vi "Initialize camera.vi"() -> (2 "CUDA device ID":i32, 3 "IMAQdx Session Out":T1, 4 "TrueFrame out":i32, 6 "IMAQ camera":bool, 8 "Image reference out":T2, 10 "SLM enabled":bool=TRUE, 11 "Camera enabled":bool=TRUE, 12 "Vision error out":errorcluster, 13 "LUT path out":path, 14 "IMAQ Session Out":refnum<k11>, 15 "Camera error":errorcluster)   [LabVIEW 2009]
uses:
  <vilib>/vision/Image Controls.llb/IMAQ Image.ctl
  <vilib>/userDefined/High Color/IMAQdx.ctl
  <vilib>/vision/driver/NI_Vision_Acquisition_Software.lvlib
panel:
  in  "CUDA device ID":i32
  in  "LUT file (full path)":path
  in  "TrueFrame":i32=6
  in  "Select camera type":u16(ring)=2 items=["IMAQ (Camera Link)", "IMAQdx (firewire)", "No camera"]
  in  "SLM enabled":bool
  in  "Start":bool
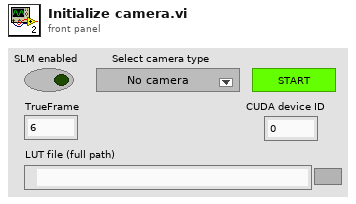
[diagram p1: front panel]
types:
  T1 = typedef "IMAQdx.ctl" = refnum<k21>
  T2 = typedef "IMAQ Image.ctl" = refnum<image>
  T3 = typedef "Image Type" = u32
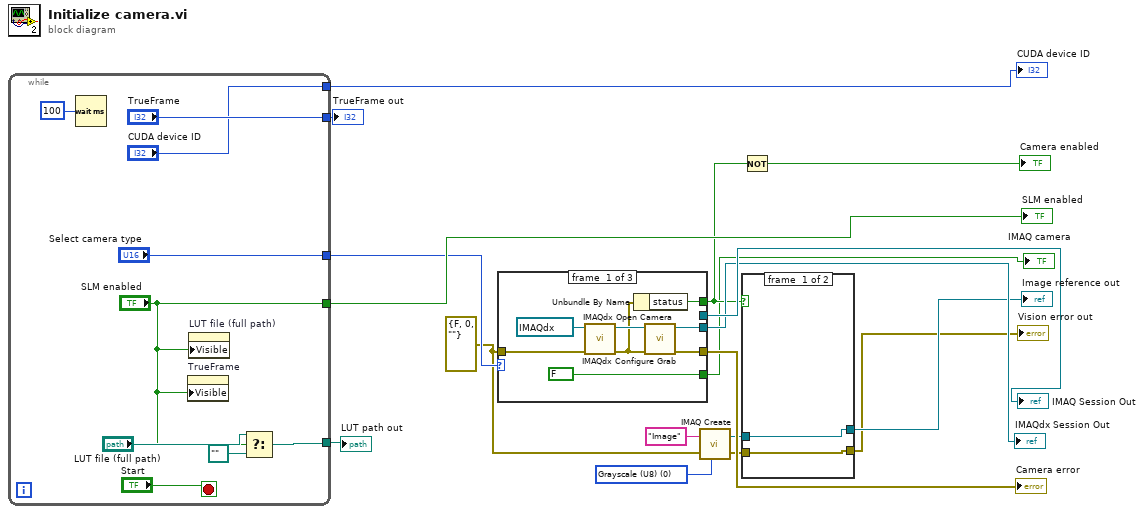
[diagram p0: block diagram]
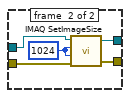
[diagram p2: hidden frame]
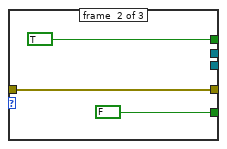
[diagram p3: hidden frame]
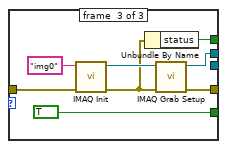
[diagram p4: hidden frame]
diagram:
  w8 = T3 0 items=["Grayscale (U8)", "Grayscale (I16)", "Grayscale (SGL)", "Complex (CSG)", "RGB (U32)", "HSL (U32)", "RGB (U64)", "Grayscale (U16)"] ("Image Type")
  w7 = errorcluster {"status"=FALSE, "code"=0, "source"=""} ("Camera error")
  n1 = while {
    tunnel: ["SLM enabled"] -> w16
    tunnel: ["Select camera type"] -> w12
    tunnel: ["TrueFrame"] -> w3
    tunnel: [w22] -> w2
    tunnel: ["CUDA device ID"] -> w1
    stop <- "Start" stop-if-true
    n2 = Wait (ms)(milliseconds to wait=u32 100) -> ()  [unwired: 1 out]
    n3 = property on="TrueFrame" class="DigNum (strict)"("Visible"="SLM enabled") -> ()  [unwired: 2 in, 2 out]
    n4 = property on="LUT file (full path)" class="Path"("Visible"="SLM enabled") -> ()  [unwired: 2 in, 2 out]
    n5 = Select(t="LUT file (full path)", s="SLM enabled", f=path "") -> (s? t:f=w22:path)
  }
  "SLM enabled" <- w16
  "TrueFrame out" <- w3
  "LUT path out" <- w2
  "CUDA device ID" <- w1
  n6 = case shown="2, Default" w12 {
    tunnel: [_ _ w44] -> w18
    tunnel: w7 -> [w35 w38 w43]
    tunnel: [w33 _ _] -> w17
    tunnel: [w30 TRUE ("status") w41] -> w11
    tunnel: [w29 w38 w40] -> w13
    tunnel: [FALSE ("IMAQ camera") FALSE ("IMAQ camera") TRUE ("IMAQ camera")] -> w10
    frame #0 {
      n7 = call <vilib>:"IMAQdx Open Camera.vi"("error in"=w35, "Session In"=T1 "cam0") -> ("error out"=w31:errorcluster, "Session Out"=w34:T1)  [unwired: 8 in]
      n8 = Unbundle By Name(w31) -> ("status"=w30:bool)
      n9 = call <vilib>:"IMAQdx Configure Grab.vi"("error in"=w31, "Session In"=w34) -> ("error out"=w29:errorcluster, "Session Out"=w33:T1)  [unwired: 8 in]
    }
    frame #1 {
    }
    frame #2 {
      n10 = call <vilib>:"IMAQ Init.vi"("error in (no error)"=w43, "Interface Name"="img0") -> ("error out"=w42:errorcluster, "IMAQ Session Out"=w45:refnum<k11>)  [unwired: 8 out]
      n11 = Unbundle By Name(w42) -> ("status"=w41:bool)
      n12 = call <vilib>:"IMAQ Grab Setup.vi"("error in (no error)"=w42, "IMAQ Session In"=w45) -> ("error out"=w40:errorcluster, "IMAQ Session Out"=w44:refnum<k11>)  [unwired: 8 out]
    }
  }
  "IMAQ Session Out" <- w18
  "IMAQdx Session Out" <- w17
  "IMAQ camera" <- w10
  "Camera error" <- w13
  n13 = call "IMAQ Create"("Image Name"="Image", "Image Type"=w8, "error in (no error)"=w7) -> ("New Image"=w5:T2, "error out"=w6:errorcluster)  [unwired: 1 in, 1 out]
  n14 = Not(x=w11) -> (.not. x?=→"Camera enabled":bool)
  n15 = case shown="True" w11 {
    tunnel: [w48 w52] -> w15
    tunnel: [w47 w51] -> w14
    tunnel: w6 -> [w47 w50]
    tunnel: w5 -> [w48 w49]
    frame #0 {
    }
    frame #1 {
      w53 = 1024 ("X Resolution")
      n16 = call "IMAQ SetImageSize"("error in (no error)"=w50, "Y Resolution"=w53, "X Resolution"=w53, "Image"=w49) -> ("error out"=w51:errorcluster, "Image Out"=w52:T2)  [unwired: 1 in]
    }
  }
  "Image reference out" <- w15
  "Vision error out" <- w14
